vi "Ke2400 Config Measure.vi"(6 "Manual Range":dbl=1.0, 8 "error in (no error)":errorcluster, 9 "Enable Auto Range?":bool, 10 "Function":u16(ring) items=["VOLT", "CURR", "RES"], 11 "VISA resource name":refnum<visa-resource-name>) -> (0 "error out":errorcluster, 3 "VISA resource name out":refnum<visa-resource-name>)   [LabVIEW 2012]
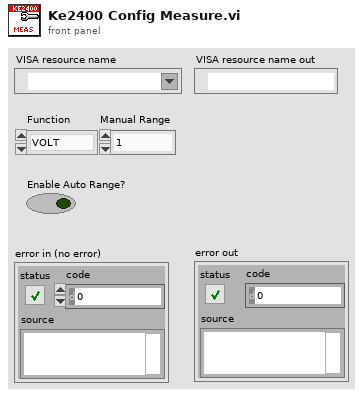
[diagram p1: front panel]
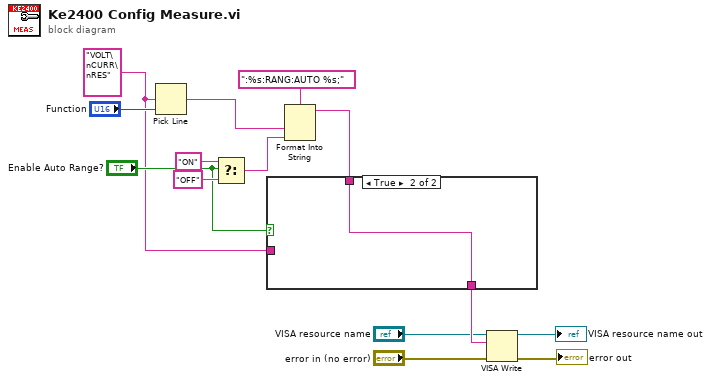
[diagram p0: block diagram]
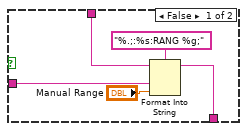
[diagram p2: hidden frame]
diagram:
  w6 = "VOLT\nCURR\nRES" ("multi-line string")
  n1 = Pick Line(multi-line string=w6, line index="Function") -> (output string=w1:string)  [unwired: 1 in]
  n2 = Select(t="ON" ("format string"), s="Enable Auto Range?", f="OFF") -> (s? t:f=w10:string)
  n3 = Format Into String(format string=":%s:RANG:AUTO %s;", w1, w10) -> (resulting string=w8:string)  [unwired: 2 in, 1 out]
  n4 = case shown="True" "Enable Auto Range?" {
    tunnel: w8 -> [w19 w20]
    tunnel: [w18 w20] -> w7
    tunnel: w6 -> [w17 _]
    frame False {
      n5 = Format Into String(format string="%.;:%s:RANG %g;", initial string=w19, w17, "Manual Range") -> (resulting string=w18:string)  [unwired: 1 in, 1 out]
    }
    frame True {
    }
  }
  n6 = VISA Write(VISA resource name="VISA resource name", write buffer=w7, error in (no error)="error in (no error)") -> (VISA resource name out=→"VISA resource name out":refnum<visa-resource-name>, error out=→"error out":errorcluster)  [unwired: 1 out]
